vi "myRIO v1.0 Read Encoder.vi"(8 "error in (no error)":errorcluster, 9 "Reset Counter":bool, 10 "Channel":T2, 11 "myRIO Ref In":T3) -> (0 "error out":errorcluster, 1 "Counter Direction":T1, 2 "Counter Value":i32, 3 "myRIO Ref Out":T3, 5 "Overflow?":bool)   [LabVIEW 2021]
uses:
  <vilib>/myRIO/Common/Instrument Driver Framework/Utilities/typedefs/myRIO v1.0 Reference.ctl
  <vilib>/myRIO/Common/Instrument Driver Framework/Utilities/typedefs/Generic FPGA Reference.ctl
  <vilib>/myRIO/Common/Instrument Driver Framework/myRIO v1.0/Encoder/typedefs/Encoder Channels Enum.ctl
  <vilib>/myRIO/Common/Instrument Driver Framework/myRIO v1.0/Encoder/typedefs/Encoder Count Direction Enum.ctl
  <vilib>/myRIO/Common/Instrument Driver Framework/myRIO v1.0/Encoder/typedefs/Encoder Channels FPGA Reference.ctl
  <vilib>/rvi/errors/niLvFpgaAdjustHostInterfaceError.vi
  <vilib>/rvi/interface/nirviReadWriteControl/nirviReadWriteControl.xnode
  <vilib>/rvi/interface/Simulation/niFpgaSimulationCallBeginRW.vi
  NiFpgaLv.dll
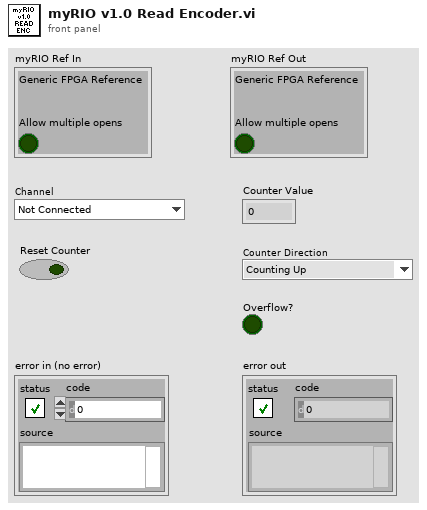
[diagram p1: front panel]
types:
  T1 = typedef "Encoder Count Direction Enum.ctl" = enum16{"Counting Up", "Counting Down"}
  T2 = typedef "Encoder Channels Enum.ctl" = enum16{"Not Connected", "C/ENC0", "C/ENC1", "A/ENC", "A/ENC0", "A/ENC1", "A/ENC2", "A/ENC3", "A/ENC4", "A/ENC5", "A/ENC6", "A/ENC7", "A/ENC8", "A/ENC9", "B/ENC", "B/ENC0", "B/ENC1", "B/ENC2", "B/ENC3", "B/ENC4", "B/ENC5", "B/ENC6", "B/ENC7", "B/ENC8", "B/ENC9", "DIO/ENC0", "DIO/ENC1", "DIO/ENC2", "DIO/ENC3", "DIO/ENC4"}
  T3 = typedef "myRIO v1.0 Reference.ctl" = cluster{"Generic FPGA Reference":T4, "Allow multiple opens":bool}
  T4 = typedef "Generic FPGA Reference.ctl" = refnum<k20>
  T5 = typedef "Encoder Channels FPGA Reference.ctl" = refnum<k20>
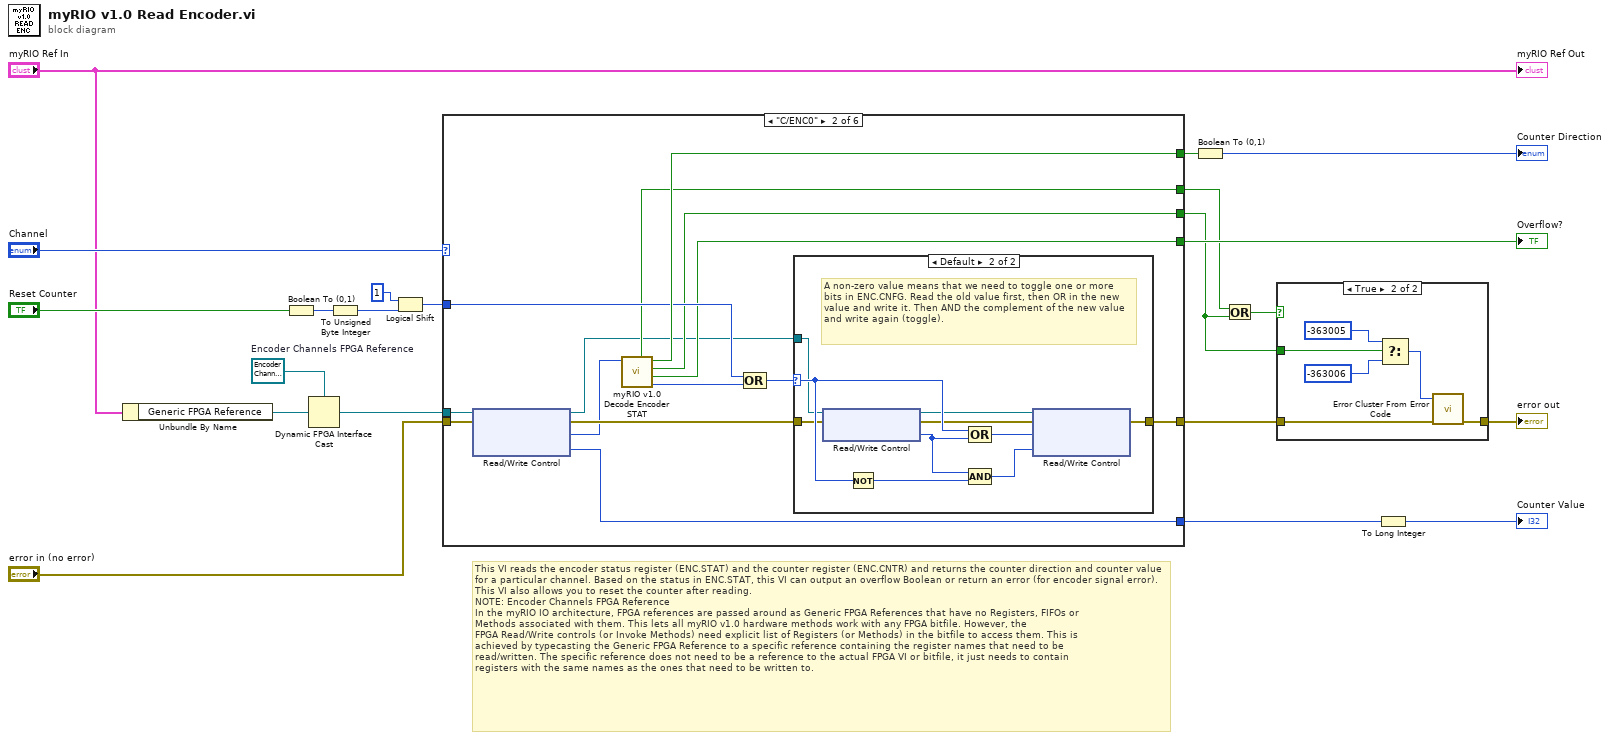
[diagram p0: block diagram]
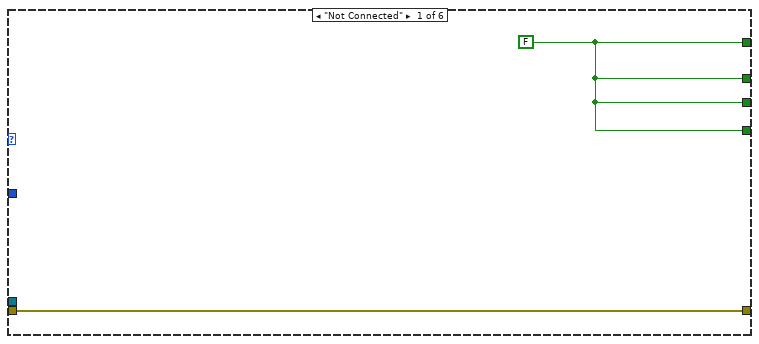
[diagram p3: hidden frame]
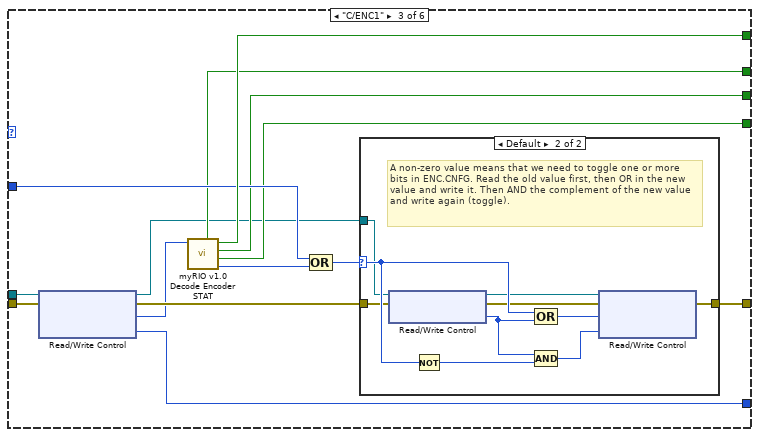
[diagram p5: hidden frame]
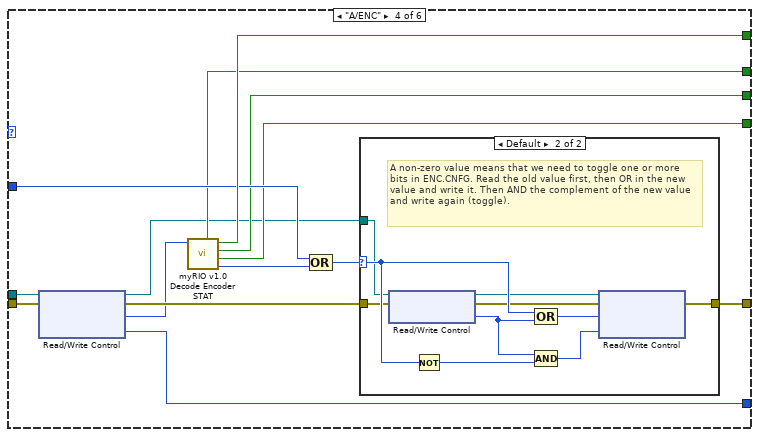
[diagram p7: hidden frame]
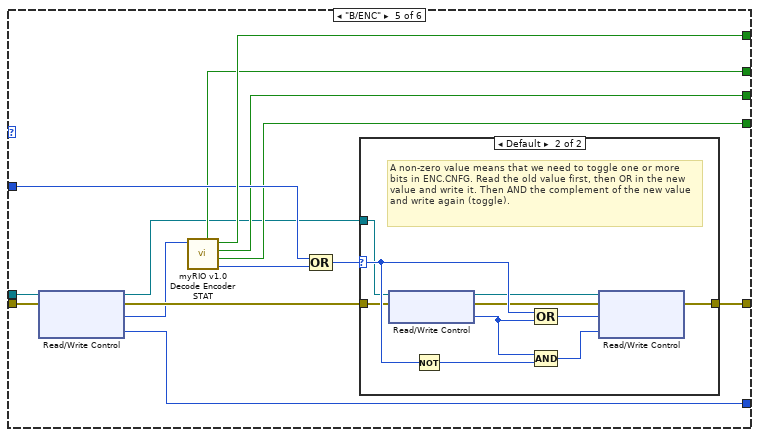
[diagram p9: hidden frame]
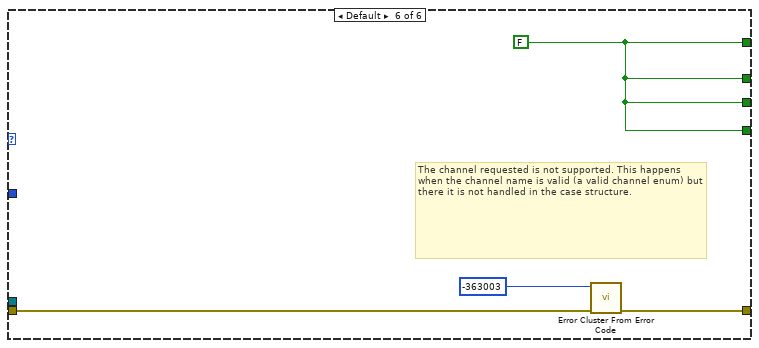
[diagram p11: hidden frame]
diagram:
  w21 = T5 refnum  # Encoder Channels FPGA Reference
  # "This VI reads the encoder status register (ENC.STAT) and the counter register (ENC.CNTR) and returns the counter direction and counter value for a particular channel. Based on the status in ENC.STAT, this VI can output an overflow Boolean or return an error (for encoder signal error). This VI also allows you to reset the counter after reading.\nNOTE: Encoder Channels FPGA Reference\nIn the myRIO IO architecture, FPGA references are passed around as Generic FPGA References that have no Registers, FIFOs or\nMethods associated with them. This lets all myRIO v1.0 hardware methods work with any FPGA bitfile. However, the \nFPGA Read/Write controls (or Invoke Methods) need explicit list of Registers (or Methods) in the bitfile to access them. This is \nachieved by typecasting the Generic FPGA Reference to a specific reference containing the register names that need to be \nread/written. The specific reference does not need to be a reference to the actual FPGA VI or bitfile, it just needs to contain \nregisters with the same names as the ones that need to be written to."
  n1 = Unbundle By Name("myRIO Ref In") -> ("Generic FPGA Reference"=w6:T4)
  n2 = Boolean To (0,1)(Boolean="Reset Counter") -> (0, 1=w7:i16)
  n3 = Dynamic FPGA Interface Cast(Session In=w21, Type=w6) -> (Session Out=w20:T5)
  n4 = To Unsigned Byte Integer(number=w7) -> (unsigned 8bit integer=w8:u8)
  n5 = Logical Shift(y=u8 1, x=w8) -> (x << y=w11:u8)
  n6 = case shown="\"C/ENC0\"" "Channel" {
    tunnel: "error in (no error)" -> [w23 w28 w53 w78 w103 w125]
    tunnel: [w23 w37 w62 w87 w112 w126] -> w16
    tunnel: w20 -> [_ w29 w54 w79 w104 _]
    tunnel: [w22 w34 w59 w84 w109 w124] -> w13
    tunnel: [_ w24 w49 w74 w99 _] -> w17
    tunnel: w11 -> [_ w33 w58 w83 w108 _]
    tunnel: [w22 w32 w57 w82 w107 w124] -> w1
    tunnel: [w22 w31 w56 w81 w106 w124] -> w9
    tunnel: [w22 w30 w55 w80 w105 w124] -> w3
    frame "Not Connected" {
      w22 = FALSE ("Counting down?")
    }
    frame "C/ENC0" {
      n7 = xnode "Read/Write Control"("FPGA VI Reference In"=w29, "error in"=w28) -> ("FPGA VI Reference Out"=w27:T5, "error out"=w26:errorcluster, "ENC.C_0.STAT"=w25:u8, "ENC.C_0.CNTR"=w24:u32)
      n8 = call <vilib>:"myRIO v1.0 Decode Encoder STAT.vi"("ENC.STAT"=w25) -> ("ENC.CNFG to write"=w35:u8, "Signed Overflow?"=w31:bool, "Error?"=w32:bool, "Counting down?"=w34:bool, "Signed Overflow Error?"=w30:bool)  [unwired: 6 in]
      n9 = Compound Arithmetic op=OR(w33, w35) -> (w36:u8)
      n10 = case shown="Default" w36 {
        selector: w36 -> [_ w47]
        tunnel: w27 -> [_ w46]
        tunnel: w26 -> [w38 w45]
        tunnel: [w38 w39] -> w37
        frame 0 {
        }
        frame Default {
          # "A non-zero value means that we need to toggle one or more bits in ENC.CNFG. Read the old value first, then OR in the new value and write it. Then AND the complement of the new value and write again (toggle)."
          n11 = xnode "Read/Write Control"("FPGA VI Reference In"=w46, "error in"=w45) -> ("FPGA VI Reference Out"=w43:T5, "error out"=w42:errorcluster, "ENC.C_0.CNFG"=w44:u8)
          n12 = Not(x=w47) -> (.not. x?=w48:u8)
          n13 = Compound Arithmetic op=OR(w47, w44) -> (w41:u8)
          n14 = Compound Arithmetic op=AND(w44, w48) -> (w40:u8)
          n15 = xnode "Read/Write Control"("FPGA VI Reference In"=w43, "error in"=w42, "ENC.C_0.CNFG"=w41, "ENC.C_0.CNFG"=w40) -> ("error out"=w39:errorcluster)  [unwired: 1 out]
        }
      }
    }
    frame "C/ENC1" {
      n16 = xnode "Read/Write Control"("FPGA VI Reference In"=w54, "error in"=w53) -> ("FPGA VI Reference Out"=w52:T5, "error out"=w51:errorcluster, "ENC.C_1.STAT"=w50:u8, "ENC.C_1.CNTR"=w49:u32)
      n17 = call <vilib>:"myRIO v1.0 Decode Encoder STAT.vi"("ENC.STAT"=w50) -> ("ENC.CNFG to write"=w60:u8, "Signed Overflow?"=w56:bool, "Error?"=w57:bool, "Counting down?"=w59:bool, "Signed Overflow Error?"=w55:bool)  [unwired: 6 in]
      n18 = Compound Arithmetic op=OR(w58, w60) -> (w61:u8)
      n19 = case shown="Default" w61 {
        selector: w61 -> [_ w72]
        tunnel: w52 -> [_ w71]
        tunnel: w51 -> [w63 w70]
        tunnel: [w63 w64] -> w62
        frame 0 {
        }
        frame Default {
          # "A non-zero value means that we need to toggle one or more bits in ENC.CNFG. Read the old value first, then OR in the new value and write it. Then AND the complement of the new value and write again (toggle)."
          n20 = xnode "Read/Write Control"("FPGA VI Reference In"=w71, "error in"=w70) -> ("FPGA VI Reference Out"=w68:T5, "error out"=w67:errorcluster, "ENC.C_1.CNFG"=w69:u8)
          n21 = Not(x=w72) -> (.not. x?=w73:u8)
          n22 = Compound Arithmetic op=OR(w72, w69) -> (w66:u8)
          n23 = Compound Arithmetic op=AND(w69, w73) -> (w65:u8)
          n24 = xnode "Read/Write Control"("FPGA VI Reference In"=w68, "error in"=w67, "ENC.C_1.CNFG"=w66, "ENC.C_1.CNFG"=w65) -> ("error out"=w64:errorcluster)  [unwired: 1 out]
        }
      }
    }
    frame "A/ENC" {
      n25 = xnode "Read/Write Control"("FPGA VI Reference In"=w79, "error in"=w78) -> ("FPGA VI Reference Out"=w77:T5, "error out"=w76:errorcluster, "ENC.A.STAT"=w75:u8, "ENC.A.CNTR"=w74:u32)
      n26 = call <vilib>:"myRIO v1.0 Decode Encoder STAT.vi"("ENC.STAT"=w75) -> ("ENC.CNFG to write"=w85:u8, "Signed Overflow?"=w81:bool, "Error?"=w82:bool, "Counting down?"=w84:bool, "Signed Overflow Error?"=w80:bool)  [unwired: 6 in]
      n27 = Compound Arithmetic op=OR(w83, w85) -> (w86:u8)
      n28 = case shown="Default" w86 {
        selector: w86 -> [_ w97]
        tunnel: w77 -> [_ w96]
        tunnel: w76 -> [w88 w95]
        tunnel: [w88 w89] -> w87
        frame 0 {
        }
        frame Default {
          # "A non-zero value means that we need to toggle one or more bits in ENC.CNFG. Read the old value first, then OR in the new value and write it. Then AND the complement of the new value and write again (toggle)."
          n29 = xnode "Read/Write Control"("FPGA VI Reference In"=w96, "error in"=w95) -> ("FPGA VI Reference Out"=w93:T5, "error out"=w92:errorcluster, "ENC.A.CNFG"=w94:u8)
          n30 = Not(x=w97) -> (.not. x?=w98:u8)
          n31 = Compound Arithmetic op=OR(w97, w94) -> (w91:u8)
          n32 = Compound Arithmetic op=AND(w94, w98) -> (w90:u8)
          n33 = xnode "Read/Write Control"("FPGA VI Reference In"=w93, "error in"=w92, "ENC.A.CNFG"=w91, "ENC.A.CNFG"=w90) -> ("error out"=w89:errorcluster)  [unwired: 1 out]
        }
      }
    }
    frame "B/ENC" {
      n34 = xnode "Read/Write Control"("FPGA VI Reference In"=w104, "error in"=w103) -> ("FPGA VI Reference Out"=w102:T5, "error out"=w101:errorcluster, "ENC.B.STAT"=w100:u8, "ENC.B.CNTR"=w99:u32)
      n35 = call <vilib>:"myRIO v1.0 Decode Encoder STAT.vi"("ENC.STAT"=w100) -> ("ENC.CNFG to write"=w110:u8, "Signed Overflow?"=w106:bool, "Error?"=w107:bool, "Counting down?"=w109:bool, "Signed Overflow Error?"=w105:bool)  [unwired: 6 in]
      n36 = Compound Arithmetic op=OR(w108, w110) -> (w111:u8)
      n37 = case shown="Default" w111 {
        selector: w111 -> [_ w122]
        tunnel: w102 -> [_ w121]
        tunnel: w101 -> [w113 w120]
        tunnel: [w113 w114] -> w112
        frame 0 {
        }
        frame Default {
          # "A non-zero value means that we need to toggle one or more bits in ENC.CNFG. Read the old value first, then OR in the new value and write it. Then AND the complement of the new value and write again (toggle)."
          n38 = xnode "Read/Write Control"("FPGA VI Reference In"=w121, "error in"=w120) -> ("FPGA VI Reference Out"=w118:T5, "error out"=w117:errorcluster, "ENC.B.CNFG"=w119:u8)
          n39 = Not(x=w122) -> (.not. x?=w123:u8)
          n40 = Compound Arithmetic op=OR(w122, w119) -> (w116:u8)
          n41 = Compound Arithmetic op=AND(w119, w123) -> (w115:u8)
          n42 = xnode "Read/Write Control"("FPGA VI Reference In"=w118, "error in"=w117, "ENC.B.CNFG"=w116, "ENC.B.CNFG"=w115) -> ("error out"=w114:errorcluster)  [unwired: 1 out]
        }
      }
    }
    frame Default {
      w124 = FALSE ("Counting down?")
      # "The channel requested is not supported. This happens when the channel name is valid (a valid channel enum) but there it is not handled in the case structure."
      n43 = call <vilib>:"Error Cluster From Error Code.vi"("error in (no error)"=w125, "error code (0)"=-363003) -> ("error out"=w126:errorcluster)  [unwired: 7 in]
    }
  }
  "Overflow?" <- w9
  n44 = Boolean To (0,1)(Boolean=w13) -> (0, 1=→"Counter Direction":i16)
  n45 = Or(x=w3, y=w1) -> (x .or. y?=w2:bool)
  n46 = case shown="True" w2 {
    tunnel: w16 -> [w128 w133]
    tunnel: [w128 w134] -> w15
    tunnel: w1 -> [_ w132]
    frame False {
    }
    frame True {
      n47 = Select(t=-363005 ("error code (0)"), s=w132, f=-363006 ("error code (0)")) -> (s? t:f=w130:i32)
      n48 = call <vilib>:"Error Cluster From Error Code.vi"("error in (no error)"=w133, "error code (0)"=w130) -> ("error out"=w134:errorcluster)  [unwired: 7 in]
    }
  }
  "error out" <- w15
  n49 = To Long Integer(number=w17) -> (32bit integer=→"Counter Value":i32)
  "myRIO Ref Out" <- "myRIO Ref In"
